vi "Collect and Analyze Warm-Up Data.vi"(5 "error in (no error)":errorcluster, 6 "Range of Readings(time)":T3 {"Lower Range" format="%.2f"; "Upper Range" format="%.2f"}, 7 "Reference":dbl format="%.2f", 8 "refnum":refnum<file>) -> (0 "error out":errorcluster, 1 "DataSets":T2 {"Deltas(PPM)" format="%.8f"; "Frequency(Hz)" format="%.2f"; "Time" format="%.2f"}, 3 "Header":T1 {"Nom Freq(MHz)" format="%.2f"; "Initial Frequency (Hz)" format="%.4f"})   [LabVIEW 2021]
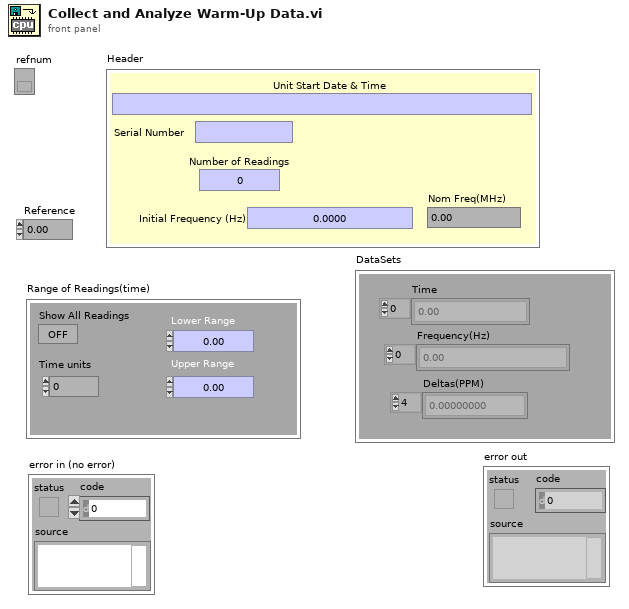
[diagram p1: front panel]
types:
  T1 = cluster{"Serial Number":string, "Number of Readings":i32, "Initial Frequency (Hz)":dbl, "Unit Start Date & Time":string, "Nom Freq(MHz)":dbl}
  T2 = cluster{"Time":dbl[], "Frequency(Hz)":dbl[], "Deltas(PPM)":dbl[]}
  T3 = cluster{"Show All Readings":bool, "Upper Range":dbl, "Lower Range":dbl, "Time units":u8}
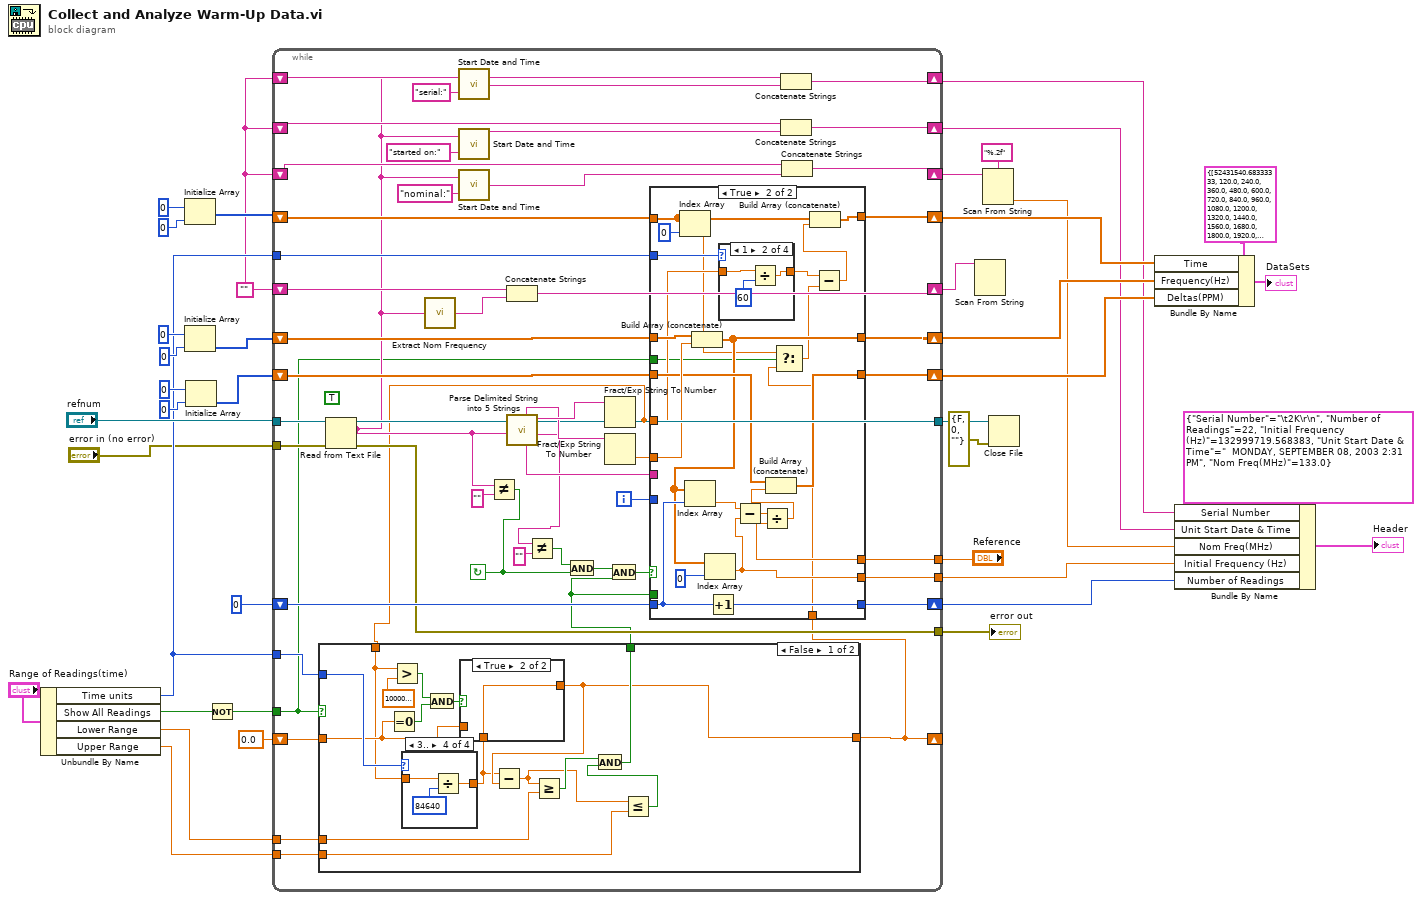
[diagram p0: block diagram]
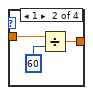
[diagram p4: hidden frame]
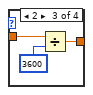
[diagram p5: hidden frame]
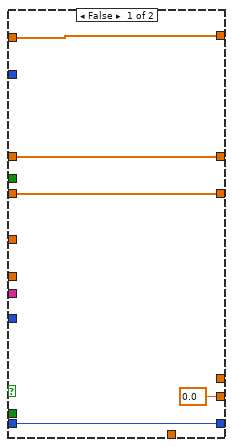
[diagram p7: hidden frame]
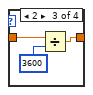
[diagram p9: hidden frame]
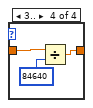
[diagram p10: hidden frame]
diagram:
  w7 = ""
  n1 = Unbundle By Name("Range of Readings(time)") -> ("Time units"=w16:u8, "Show All Readings"=w17:bool, "Lower Range"=w15:dbl, "Upper Range"=w14:dbl)
  n2 = Initialize Array(0, 0) -> (w30:i32[])
  n3 = Initialize Array(0, 0) -> (w29:i32[])
  n4 = Initialize Array(0, 0) -> (w37:i32[])
  n5 = Not(x=w17) -> (.not. x?=w1:bool)
  n6 = while {
    shift-left: w7 -> [w72]
    shift-right: [w70] -> w27
    shift-left: 0.0 -> [w73]
    shift-right: [w43] -> _
    tunnel: w16 -> [w74]
    tunnel: "Reference" -> [w78]
    tunnel: w16 -> [w79]
    shift-left: 0 -> [w81]
    shift-right: [w80] -> w9
    shift-left: w37 -> [w83]
    shift-right: [w82] -> w20
    shift-left: w29 -> [w86]
    shift-right: [w88] -> w19
    shift-left: w30 -> [w87]
    shift-right: [w42] -> w21
    tunnel: "refnum" -> [w64]
    tunnel: [w63] -> w25
    shift-right: [w62] -> w11
    shift-left: w7 -> [w61]
    tunnel: w1 -> [w40]
    tunnel: w14 -> [w59]
    tunnel: w15 -> [w58]
    tunnel: [w57] -> w8
    shift-right: [w54] -> w10
    shift-left: w7 -> [w53]
    shift-right: [w50] -> w6
    shift-left: w7 -> [w48]
    tunnel: "error in (no error)" -> [w46]
    tunnel: [w45] -> w2
    i -> [w65]
    stop <- w77 continue-if-true
    (unwired) TRUE ("line mode (F)")
    n7 = Read from Text File(file (use dialog)=w64, error in=w46) -> (refnum out=w63:refnum<file>, text=w47:string, error out=w45:errorcluster)  [unwired: 2 in, 1 out]
    n8 = call "Extract Nom Frequency.vi"("String to Parse"=w47) -> ("Nominal Frequency"=w71:string)
    n9 = call "Start Date and Time.vi"("Search Detail"="serial:", "String IN"=w47) -> ("Header Detail"=w52:string)
    n10 = call "Start Date and Time.vi"("Search Detail"="started on:", "String IN"=w47) -> ("Header Detail"=w60:string)
    n11 = call "Start Date and Time.vi"("Search Detail"="nominal:", "String IN"=w47) -> ("Header Detail"=w49:string)
    n12 = Not Equal?(x=w47, y="") -> (x != y?=w77:bool)
    n13 = Concatenate Strings(w72, w71) -> (w70:string)
    n14 = call "Parse Delimited String into 5 Strings"("String to Parse"=w47) -> ("String 1"=w67:string, "Serial"=w69:string, "String 2"=w68:string, "String 4"=w66:string)  [unwired: 3 out]
    n15 = Not Equal?(x=w66, y="") -> (x != y?=w84:bool)
    n16 = And(x=w84, y=w77) -> (x .and. y?=w76:bool)
    n17 = Fract/Exp String To Number(string=w68) -> (number=w44:dbl)  [unwired: 3 in, 1 out]
    n18 = case shown="False" w40 {
      selector: w40 -> [_ w119]
      tunnel: [w104 w119] -> w41
      tunnel: w74 -> [w105 _]
      tunnel: w44 -> [w93 _]
      tunnel: w73 -> [w98 w118]
      tunnel: [w97 w118] -> w43
      tunnel: w59 -> [w95 _]
      tunnel: w58 -> [w94 _]
      frame False {
        n19 = Equal To 0?(x=w98) -> (x = 0?=w99:bool)
        n20 = Greater?(x=w93, y=1000000.0) -> (0:w91:bool)
        n21 = case shown="3.." w105 {
          tunnel: w93 -> [w108 w111 w114 w117]
          tunnel: [w108 w110 w113 w116] -> w96
          frame ..0 {
          }
          frame 1 {
            n22 = Divide(x=w111, y=60) -> (x/y=w110:dbl)
          }
          frame 2 {
            n23 = Divide(x=w114, y=3600) -> (x/y=w113:dbl)
          }
          frame 3.. {
            n24 = Divide(x=w117, y=84640) -> (x/y=w116:dbl)
          }
        }
        n25 = And(x=w91, y=w99) -> (x .and. y?=w100:bool)
        n26 = case shown="True" w100 {
          tunnel: [w106 w107] -> w97
          tunnel: w98 -> [w106 _]
          tunnel: w96 -> [_ w107]
          frame False {
          }
          frame True {
          }
        }
        n27 = Subtract(x=w96, y=w97) -> (x-y=w101:dbl)
        n28 = Greater Or Equal?(x=w101, y=w94) -> (x >= y?=w103:bool)
        n29 = Less Or Equal?(x=w101, y=w95) -> (x <= y?=w102:bool)
        n30 = And(x=w103, y=w102) -> (x .and. y?=w104:bool)
      }
      frame True {
      }
    }
    n31 = Fract/Exp String To Number(string=w67) -> (number=w89:dbl)  [unwired: 3 in, 1 out]
    n32 = And(x=w76, y=w41) -> (x .and. y?=w75:bool)
    n33 = case shown="True" w75 {
      tunnel: w44 -> [_ w131]
      tunnel: w89 -> [_ w147]
      tunnel: [w124 w146] -> w42
      tunnel: [w123 w136] -> w88
      tunnel: w87 -> [w124 w130]
      tunnel: w86 -> [w123 w148]
      tunnel: w83 -> [w122 w144]
      tunnel: [w122 w143] -> w82
      tunnel: w81 -> [w121 w141]
      tunnel: [w121 w142] -> w80
      tunnel: w65 -> [_ _]
      tunnel: w79 -> [_ w140]
      tunnel: w78 -> [_ w138]
      tunnel: w69 -> [_ _]
      tunnel: [0.0 w132] -> w57
      tunnel: w43 -> [_ w126]
      tunnel: w41 -> [_ _]
      tunnel: w40 -> [_ w127]
      frame False {
      }
      frame True {
        n34 = Index Array(array=w130, index=0) -> (element=w125:dbl)
        n35 = Build Array (concatenate)(w148, w147) -> (w136:dbl[])
        n36 = Index Array(array=w136, index=w141) -> (element=w145:dbl)
        n37 = Index Array(array=w136, index=0) -> (element=w132:dbl)
        n38 = Increment(x=w141) -> (x+1=w142:i32)
        n39 = case shown="1" w140 {
          tunnel: w131 -> [w149 w152 w155 w158]
          tunnel: [w149 w151 w154 w157] -> w134
          frame ..0 {
          }
          frame 1 {
            n40 = Divide(x=w152, y=60) -> (x/y=w151:dbl)
          }
          frame 2 {
            n41 = Divide(x=w155, y=3600) -> (x/y=w154:dbl)
          }
          frame 3.. {
            n42 = Divide(x=w158, y=84640) -> (x/y=w157:dbl)
          }
        }
        n43 = Subtract(x=w145, y=w132) -> (x-y=w139:dbl)
        n44 = Divide(x=w139, y=w138) -> (x/y=w137:dbl)
        n45 = Build Array (concatenate)(w144, w137) -> (w143:dbl[])
        n46 = Select(t=w125, s=w127, f=w126) -> (s? t:f=w129:dbl)
        n47 = Subtract(x=w134, y=w129) -> (x-y=w133:dbl)
        n48 = Build Array (concatenate)(w130, w133) -> (w146:dbl[])
      }
    }
    n49 = Concatenate Strings(w53, w52) -> (w54:string)
    n50 = Concatenate Strings(w61, w60) -> (w62:string)
    n51 = Concatenate Strings(w48, w49) -> (w50:string)
  }
  "error out" <- w2
  n52 = Scan From String(input string=w27) -> ()  [unwired: 5 in, 3 out]
  n53 = Scan From String(format string="%.2f", input string=w6) -> (output 1=w4:dbl)  [unwired: 3 in, 3 out]
  n54 = Close File(refnum=w25, error in=errorcluster {"status"=FALSE, "code"=0, "source"=""}) -> ()  [unwired: 2 out]
  n55 = Bundle By Name(cluster=T2 {"Time"=[52431540.68333333, 120.0, 240.0, 360.0, 480.0, 600.0, 720.0, 840.0, 960.0, 1080.0, 1200.0, 1320.0, 1440.0, 1560.0, 1680.0, 1800.0, 1920.0, 2040.0, 2160.0, 2280.0, 2400.0, 2520.0], "Frequency(Hz)"=[132999719.568383, 132999724.492942, 132999727.415854, 132999729.267, 132999728.656253, 132999737.993672, 132999739.268168, 132999730.419144, 132999734.663931, 132999733.339923, 132999732.443398, 132999734.312821, 132999733.825765, 132999735.028915, 132999733.812691, 132999734.524936, 132999740.046434, 132999732.262498, 132999732.75918, 132999734.256276, 132999735.296532, 132999734.67656], "Deltas(PPM)"=[0.0, 37.02675948913832, 59.00354145612931, 72.92193241585466, 68.32984963754066, 138.53600755670016, 148.11868427839494, 81.58466925746515, 113.50036093166895, 103.54541354161455, 96.80462410127309, 110.86043614642064, 107.19836094325646, 116.24460157595182, 107.10006022363676, 112.4552858055086, 153.9703083217592, 95.44447378108376, 99.1789248204769, 110.43528573853628, 118.25675948670035, 113.59531583642601]} ("DataSets"), "Time"=w21, "Frequency(Hz)"=w19, "Deltas(PPM)"=w20) -> (→"DataSets":T2)
  n56 = Bundle By Name(cluster=T1 {"Serial Number"="\t2K\r\n", "Number of Readings"=22, "Initial Frequency (Hz)"=132999719.568383, "Unit Start Date & Time"="  MONDAY, SEPTEMBER 08, 2003 2:31 PM", "Nom Freq(MHz)"=133.0} ("Header"), "Serial Number"=w10, "Unit Start Date & Time"=w11, "Nom Freq(MHz)"=w4, "Initial Frequency (Hz)"=w8, "Number of Readings"=w9) -> (→"Header":T1)
